vi "Recursive Add Child Classes to Test Case Set.vi"(8 "error in (no error)":errorcluster, 10 "LVClassLibrary Refnum":refnum<vi>, 11 "Icon Decorator in":refnum<class "Icon Decorator.lvclass">) -> (0 "error out":errorcluster, 3 "Icon Decorator out":refnum<class "Icon Decorator.lvclass">)   [LabVIEW 2020, in "Icon Decorator.lvclass"]
uses:
  Icon Decorator.lvclass
  Icon Decorator.lvclass/Icon Decorator.ctl
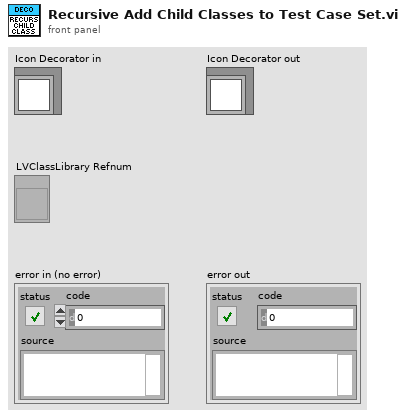
[diagram p1: front panel]
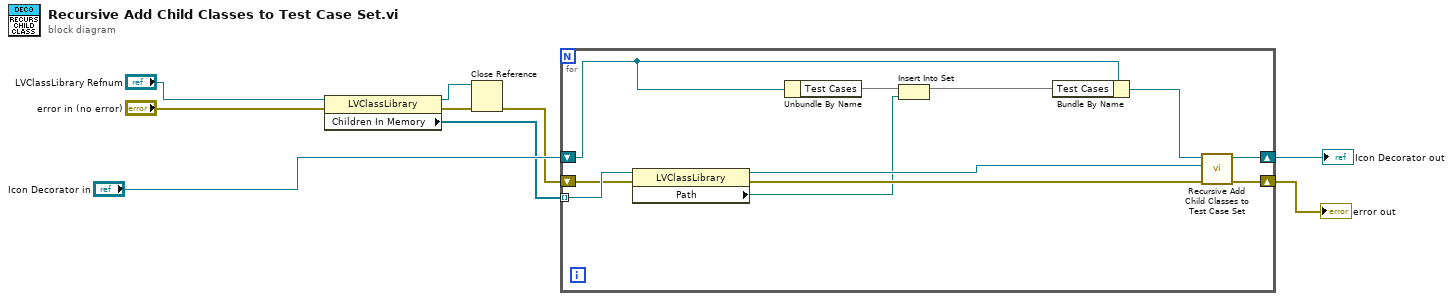
[diagram p0: block diagram]
diagram:
  n1 = property class="LVClassLibrary"(reference="LVClassLibrary Refnum", error in="error in (no error)") -> (reference out=w1:refnum<vi>, error out=w3:errorcluster, "Children In Memory"=w4:refnum<vi>[])
  n2 = Close Reference(reference=w1, error in (no error)=w3) -> (error out=w2:errorcluster)
  n3 = for {
    tunnel: w4 -> [w15] mode=indexing
    shift-right: [w18] -> w6
    shift-left: "Icon Decorator in" -> [w20]
    shift-right: [w17] -> w5
    shift-left: w2 -> [w14]
    n4 = property class="LVClassLibrary"(reference=w15, error in=w14) -> (reference out=w16:refnum<vi>, error out=w13:errorcluster, "Path"=w12:path)
    n5 = Unbundle By Name(w20) -> ("Test Cases"=w11:set{path})
    n6 = Insert Into Set(10:w12, 11:w11) -> (3:w10:set{path})  [unwired: 1 out]
    n7 = Bundle By Name(cluster=w20, "Test Cases"=w10) -> (w19:refnum<class "Icon Decorator.lvclass">)
    n8 = call "Recursive Add Child Classes to Test Case Set.vi"("error in (no error)"=w13, "LVClassLibrary Refnum"=w16, "Icon Decorator in"=w19) -> ("error out"=w17:errorcluster, "Icon Decorator out"=w18:refnum<class "Icon Decorator.lvclass">)  [unwired: 7 in]
  }
  "Icon Decorator out" <- w6
  "error out" <- w5
